vi "Check Events.vi"(8 "error in (no error)":errorcluster, 11 "GUI Helper in":refnum<class "GUI Helper.lvclass">) -> (0 "error out":errorcluster, 3 "GUI Helper out":refnum<class "GUI Helper.lvclass">)   [LabVIEW 2020, in "VolatusGUI.lvlib" / "GUI Helper.lvclass"]
uses:
  GUI Helper.lvclass
  GUI Helper.lvclass/GUI Helper.ctl
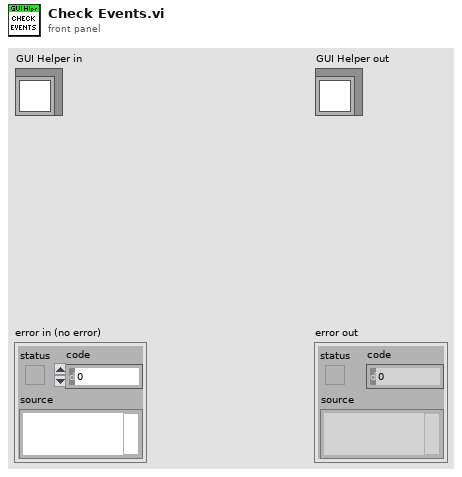
[diagram p1: front panel]
types:
  T1 = enum32{"Invalid", "Standard", "Closed", "Hidden", "Minimized", "Maximized"}
  T2 = typedef "LVRectTypeDef.ctl" = cluster{"Left":i16, "Top":i16, "Right":i16, "Bottom":i16}
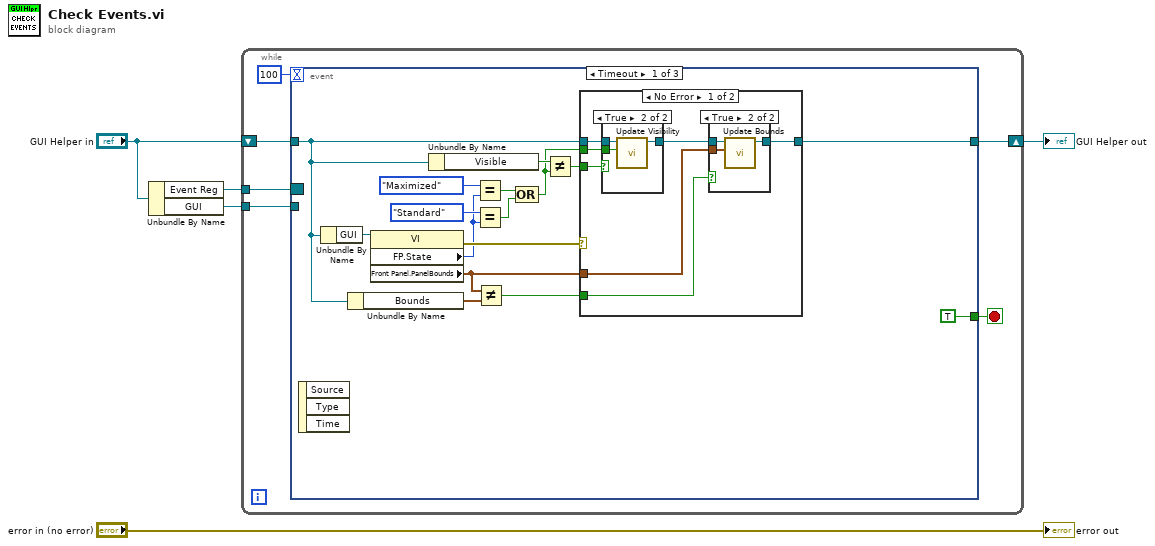
[diagram p0: block diagram]
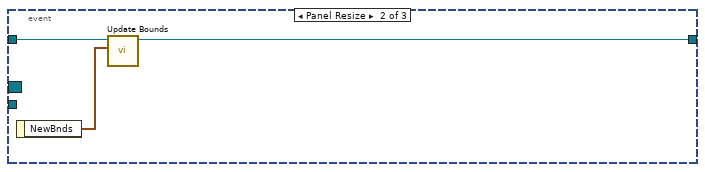
[diagram p5: hidden frame]
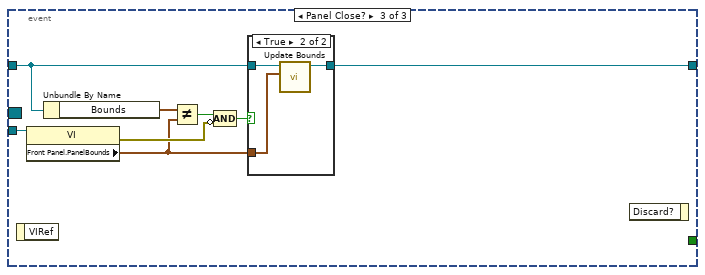
[diagram p6: hidden frame]
diagram:
  n1 = Unbundle By Name("GUI Helper in") -> ("Event Reg"=w3:refnum<event-registration>, "GUI"=w2:refnum<vi>)
  n2 = while {
    shift-right: [w8] -> w5
    shift-left: "GUI Helper in" -> [w10]
    tunnel: w3 -> [w7]
    tunnel: w2 -> [w6]
    stop <- w9 stop-if-true
    n3 = event shown="[0] Timeout" {
      selector: w7 -> [_ _ _]
      dyn-events: _ -> [_ _ _]
      timeout: 100 -> [_ _ _]
      tunnel: w10 -> [w17 w46 w50]
      tunnel: [TRUE _ _] -> w9
      tunnel: [w12 w45 w51] -> w8
      tunnel: w6 -> [_ _ w53]
      event Timeout {
        n4 = event-data() -> ()  [unwired: 1 in, 3 out]
        n5 = Unbundle By Name(w17) -> ("GUI"=w25:refnum<vi>)
        n6 = Unbundle By Name(w17) -> ("Bounds"=w19:T2)
        n7 = property class="VI"(reference=w25) -> (error out=w27:errorcluster, "FP.State"=w22:T1, "Front Panel.PanelBounds"=w13:T2)  [unwired: 1 in, 1 out]
        n8 = Unbundle By Name(w17) -> ("Visible"=w18:bool)
        n9 = Equal?(x=T1."Maximized", y=w22) -> (x = y?=w21:bool)
        n10 = Equal?(x=T1."Standard", y=w22) -> (x = y?=w20:bool)
        n11 = Not Equal?(x=w13, y=w19) -> (x != y?=w14:bool)
        n12 = Compound Arithmetic op=OR(w21, w20) -> (w15:bool)
        n13 = Not Equal?(x=w18, y=w15) -> (x != y?=w16:bool)
        n14 = case shown="No Error" w27 {
          tunnel: w17 -> [w34 w43]
          tunnel: w16 -> [w33 _]
          tunnel: w15 -> [w32 _]
          tunnel: w14 -> [w30 _]
          tunnel: w13 -> [w29 _]
          tunnel: [w28 w43] -> w12
          frame No Error {
            n15 = case shown="True" w33 {
              tunnel: w34 -> [w39 w42]
              tunnel: w32 -> [_ w41]
              tunnel: [w39 w40] -> w31
              frame False {
              }
              frame True {
                n16 = call "Update Visibility.vi"("Visible"=w41, "GUI Helper in"=w42) -> ("GUI Helper out"=w40:refnum<class "GUI Helper.lvclass">)  [unwired: 8 in, 1 out]
              }
            }
            n17 = case shown="True" w30 {
              tunnel: w31 -> [w35 w38]
              tunnel: w29 -> [_ w37]
              tunnel: [w35 w36] -> w28
              frame False {
              }
              frame True {
                n18 = call "Update Bounds.vi"("Bounds"=w37, "GUI Helper in"=w38) -> ("GUI Helper out"=w36:refnum<class "GUI Helper.lvclass">)  [unwired: 8 in, 1 out]
              }
            }
          }
          frame Error {
          }
        }
      }
      event Panel Resize {
        n19 = event-data() -> ("NewBnds"=w44:T2)  [unwired: 1 in]
        n20 = call "Update Bounds.vi"("Bounds"=w44, "GUI Helper in"=w46) -> ("GUI Helper out"=w45:refnum<class "GUI Helper.lvclass">)  [unwired: 8 in, 1 out]
      }
      event Panel Close? {
        n21 = event-data() -> ()  [unwired: 1 in, 1 out]
        n22 = property class="VI"(reference=w53) -> (error out=w54:errorcluster, "Front Panel.PanelBounds"=w49:T2)  [unwired: 1 in, 1 out]
        n23 = Unbundle By Name(w50) -> ("Bounds"=w52:T2)
        n24 = Not Equal?(x=w52, y=w49) -> (x != y?=w48:bool)
        n25 = Compound Arithmetic op=AND(w48, invert w54) -> (w47:bool)
        n26 = case shown="True" w47 {
          tunnel: [w55 w58] -> w51
          tunnel: w50 -> [w55 w57]
          tunnel: w49 -> [_ w56]
          frame False {
          }
          frame True {
            n27 = call "Update Bounds.vi"("Bounds"=w56, "GUI Helper in"=w57) -> ("GUI Helper out"=w58:refnum<class "GUI Helper.lvclass">)  [unwired: 8 in, 1 out]
          }
        }
        n28 = event-data() -> ()  [unwired: 2 in, 1 out]
      }
    }
  }
  "GUI Helper out" <- w5
  "error out" <- "error in (no error)"
